vi "Set SLSC Switch Description.vi"(8 "error in (no error)":errorcluster, 10 "Description":string, 11 "SLSC Switch Custom Device Ref in":T1 format="%.0x") -> (0 "error out":errorcluster, 3 "SLSC Switch Custom Device Ref out":T1 format="%.0x")   [LabVIEW 2017, in "SLSC Switch Scripting.lvlib"]
uses:
  SLSC Switch Scripting.lvlib
  <vilib>/NI Veristand/Custom Device API/Custom Device Item Ref.ctl
  Shared/Constants.vi
  <vilib>/NI VeriStand/Custom Device API/Custom Device API.lvlib
  Shared/SLSC Switch Shared.lvlib
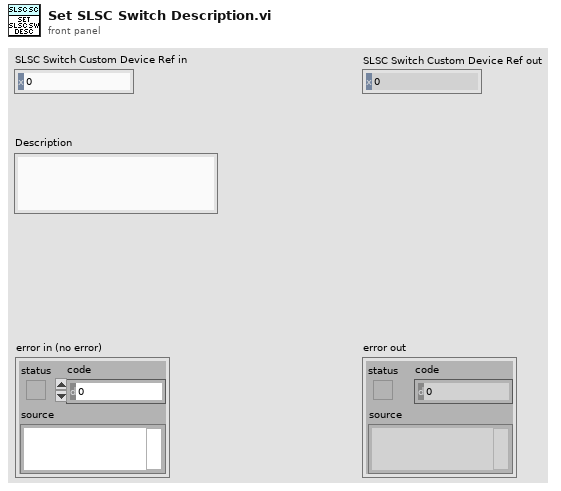
[diagram p1: front panel]
types:
  T1 = typedef "Custom Device API.lvlib/Custom Device Item Ref.ctl" = u64
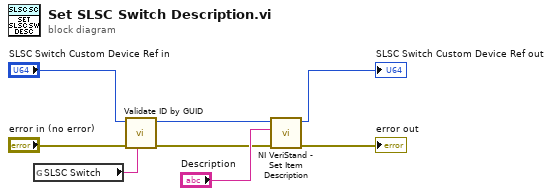
[diagram p0: block diagram]
diagram:
  n1 = global read "Constants.vi" "SLSC Switch"() -> (w2:string)
  n2 = call "Validate ID by GUID.vi"("GUID"=w2, "error in (no error)"="error in (no error)", "Ref ID in"="SLSC Switch Custom Device Ref in") -> ("error out"=w5:errorcluster, "Ref ID out"=w3:T1)  [unwired: 7 in]
  n3 = call <vilib>:"NI VeriStand - Set Item Description.vi"("error in (no error)"=w5, "Description"="Description", "Item Ref in"=w3) -> ("error out"=→"error out":errorcluster, "Item Ref out"=→"SLSC Switch Custom Device Ref out":T1)  [unwired: 6 in, 1 out]
